vi "Rotate Vector.vi"(8 "error in":errorcluster, 10 "Angle [180,-180]":dbl min=-180.0 max=180.0, 11 "PVector in":refnum<class "PVector.lvclass">) -> (0 "error out":errorcluster, 3 "PVector out":refnum<class "PVector.lvclass">)   [LabVIEW 2016, in "PVector.lvclass"]
doc: "Perform vector transformation by changing its direction while preserving its magnitude. \nThe rotation of the vector is performed using a rotational matrix: <B>V'</B> = <B>R*V</B>"
uses:
  PVector.lvclass
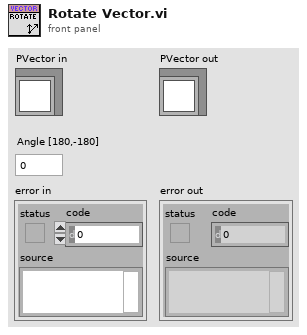
[diagram p1: front panel]
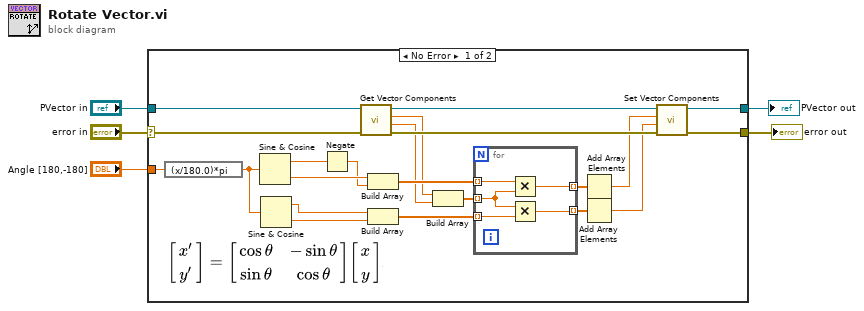
[diagram p0: block diagram]
diagram:
  n1 = case shown="No Error" "error in" {
    selector: "error in" -> [w17 w34]
    tunnel: [w16 w34] -> w4
    tunnel: [w18 w33] -> w2
    tunnel: "PVector in" -> [w20 w33]
    tunnel: "Angle [180,-180]" -> [w27 _]
    frame No Error {
      n2 = expression code="(x/180.0)*pi" ("degrees to radians")(w27) -> (w23:dbl)
      n3 = Sine & Cosine(0:w23) -> (1:w26:dbl, 2:w25:dbl)
      n4 = Sine & Cosine(0:w23) -> (1:w22:dbl, 2:w21:dbl)
      n5 = Negate(x=w26) -> (-x=w24:dbl)
      n6 = call "Get Vector Components.vi"("error in"=w17, "PVector in"=w20) -> ("error out"=w13:errorcluster, "Y"=w11:dbl, "X"=w12:dbl, "PVector out"=w19:refnum<class "PVector.lvclass">)  [unwired: 6 in]
      n7 = Build Array(w25, w24) -> (w15:dbl[])
      n8 = Build Array(w22, w21) -> (w14:dbl[])
      n9 = Build Array(w12, w11) -> (w10:dbl[])
      n10 = for {
        tunnel: w15 -> [w32] mode=indexing
        tunnel: w14 -> [w30] mode=indexing
        tunnel: w10 -> [w31] mode=indexing
        tunnel: [w29] -> w9 mode=indexing
        tunnel: [w28] -> w8 mode=indexing
        n11 = Multiply(x=w32, y=w31) -> (x*y=w29:dbl)
        n12 = Multiply(x=w31, y=w30) -> (x*y=w28:dbl)
      }
      n13 = Add Array Elements(numeric array=w9) -> (sum=w7:dbl)
      n14 = Add Array Elements(numeric array=w8) -> (sum=w6:dbl)
      n15 = call "Set Vector Components.vi"("error in"=w13, "Y"=w6, "X"=w7, "PVector in"=w19) -> ("error out"=w16:errorcluster, "PVector out"=w18:refnum<class "PVector.lvclass">)  [unwired: 6 in]
    }
    frame Error {
    }
  }
  "error out" <- w4
  "PVector out" <- w2
